vi "Read classes.vi"(8 "error in (no error)":errorcluster, 11 "S4GEI in":refnum<class "S4GEI.lvclass">) -> (0 "error out":errorcluster, 2 "classes":T1, 3 "S4GEI out":refnum<class "S4GEI.lvclass">)   [LabVIEW 2018, in "S4GEI.lvclass"]
uses:
  S4GEI.lvclass
  State Machine/State Machine.lvclass
  Channel GUI/Channel.lvclass
  RxTx/RxTx.lvclass
  S4ICS/S4ICS.lvclass
  Request/Request.lvclass
  S4GEI.lvclass/S4GEI.ctl
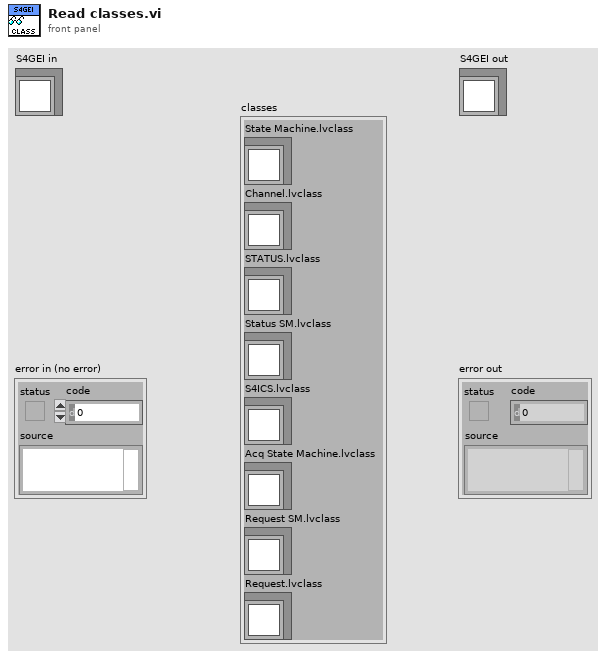
[diagram p1: front panel]
types:
  T1 = cluster{"State Machine.lvclass":refnum<class "State Machine.lvclass">, "Channel.lvclass":refnum<class "Channel.lvclass">, "STATUS.lvclass":refnum<class "RxTx.lvclass">, "Status SM.lvclass":refnum<class "State Machine.lvclass">, "S4ICS.lvclass":refnum<class "S4ICS.lvclass">, "Acq State Machine.lvclass":refnum<class "State Machine.lvclass">, "Request SM.lvclass":refnum<class "State Machine.lvclass">, "Request.lvclass":refnum<class "Request.lvclass">}
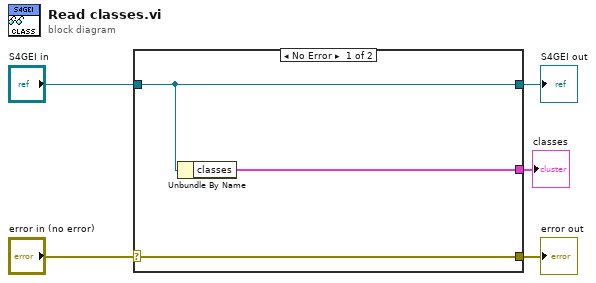
[diagram p0: block diagram]
diagram:
  n1 = case shown="No Error" "error in (no error)" {
    selector: "error in (no error)" -> [w8 w9]
    tunnel: [w8 w9] -> w4
    tunnel: [w7 w10] -> w2
    tunnel: "S4GEI in" -> [w7 w10]
    tunnel: [w6 _] -> w1
    frame No Error {
      n2 = Unbundle By Name(w7) -> ("classes"=w6:T1)
    }
    frame Error {
    }
  }
  "error out" <- w4
  "S4GEI out" <- w2
  "classes" <- w1
